vi "Serial_Write_Read_concat_Labview Community Ed.vi"() -> ()   [LabVIEW 2023]
uses:
  <vilib>/Instr/_visa.llb/VISA Configure Serial Port (Instr).vi
panel:
  in  "error in (no error)":errorcluster
  in  "byte count\nRead":u32
  in  "Number 2":u32
  in  "Number 1":u32
  in  "Loop Timer":u32
  out "Concatenated \nNumber":string
  in  "baud rate (9600)":u32=9600
  in  "VISA resource name":refnum<visa-resource-name>
  in  "stop":bool
  out "byte count Sent":u32
  out "read buffer":string
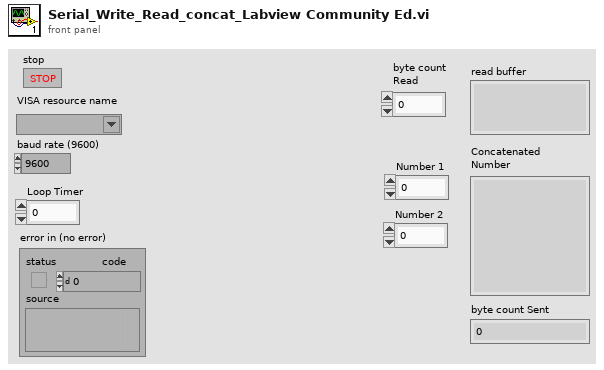
[diagram p1: front panel]
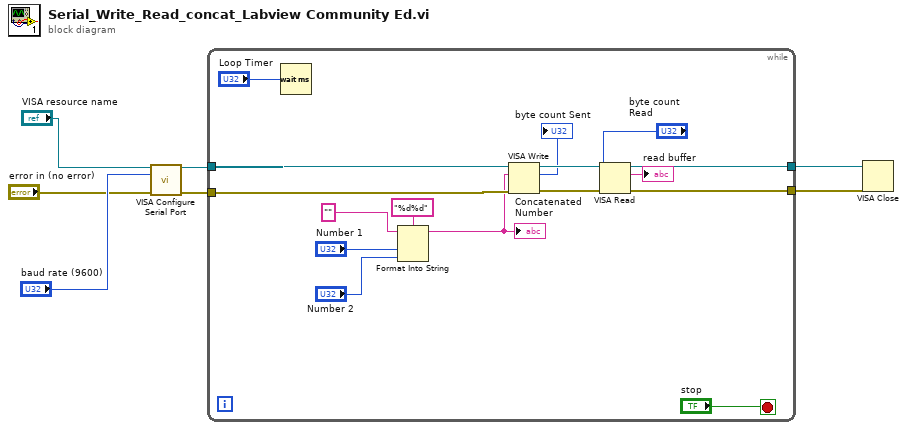
[diagram p0: block diagram]
diagram:
  n1 = call-poly "VISA Configure Serial Port"("VISA resource name"="VISA resource name", "baud rate (9600)"="baud rate (9600)", "error in (no error)"="error in (no error)") -> ("VISA resource name out"=w5:refnum<visa-resource-name>, "error out"=w4:errorcluster)  [unwired: 11 in]
  n2 = while {
    tunnel: [w22] -> w7
    tunnel: [w20] -> w6
    tunnel: w5 -> [w17]
    tunnel: w4 -> [w16]
    stop <- "stop" stop-if-true
    n3 = Wait (ms)(milliseconds to wait="Loop Timer") -> ()  [unwired: 1 out]
    n4 = Format Into String(format string="%d%d", initial string="", "Number 1", "Number 2") -> (resulting string=w10:string)  [unwired: 1 in, 1 out]
    "Concatenated \nNumber" <- w10
    n5 = VISA Write(VISA resource name=w17, write buffer=w10, error in (no error)=w16) -> (VISA resource name out=w23:refnum<visa-resource-name>, return count=→"byte count Sent":u32, error out=w19:errorcluster)
    n6 = VISA Read(VISA resource name=w23, byte count="byte count\nRead", error in (no error)=w19) -> (VISA resource name out=w22:refnum<visa-resource-name>, read buffer=→"read buffer":string, error out=w20:errorcluster)  [unwired: 1 out]
  }
  n7 = VISA Close(VISA resource name=w7, error in (no error)=w6) -> ()  [unwired: 1 out]
